vi "Read Test Group Database.vi"(8 "error in (no error)":errorcluster, 11 "Test Group Manager in":refnum<class "Test Group Manager.lvclass">) -> (0 "error out":errorcluster, 2 "Test Group Database":variant, 3 "Test Group Manager out":refnum<class "Test Group Manager.lvclass">)   [LabVIEW 2016, in "Test Group Manager.lvlib" / "Test Group Manager.lvclass"]
uses:
  Test Group Manager.lvclass
  Test Group Manager.lvclass/Test Group Manager.ctl
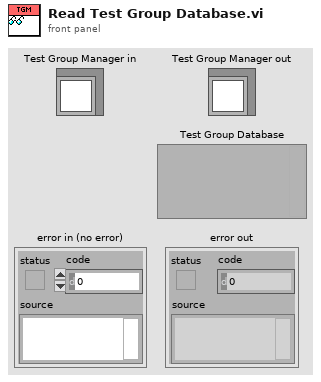
[diagram p1: front panel]
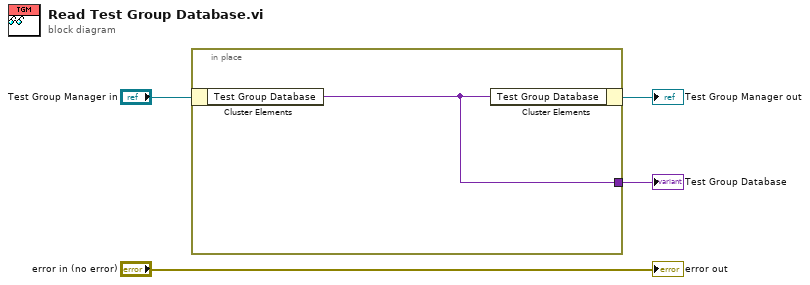
[diagram p0: block diagram]
diagram:
  n1 = in-place {
    in-place-border: [w5] -> w1
    n2 = in-place-cluster #1("Test Group Manager in") -> ("Test Group Database"=w5:variant)
    n3 = in-place-cluster #1("Test Group Database"=w5) -> (→"Test Group Manager out":refnum<class "Test Group Manager.lvclass">)
  }
  "Test Group Database" <- w1
  "error out" <- "error in (no error)"
